vi "Configure Current Limit.vi"(8 "error in (no error)":errorcluster, 10 "Current Limit":dbl, 11 "Manual PSU in":refnum<class "Manual PSU.lvclass">) -> (0 "error out":errorcluster, 3 "Manual PSU out":refnum<class "Manual PSU.lvclass">)   [LabVIEW 2020, in "Manual PSU.lvclass"]
uses:
  Manual PSU.lvclass
  C:/Sandbox/RF Bench/Source Code/WiSpry Test Framework/Instruments/Power Supply/Power Supply.lvclass
  Power Supply.lvclass/Power Supply.ctl
  Power Supply.lvclass
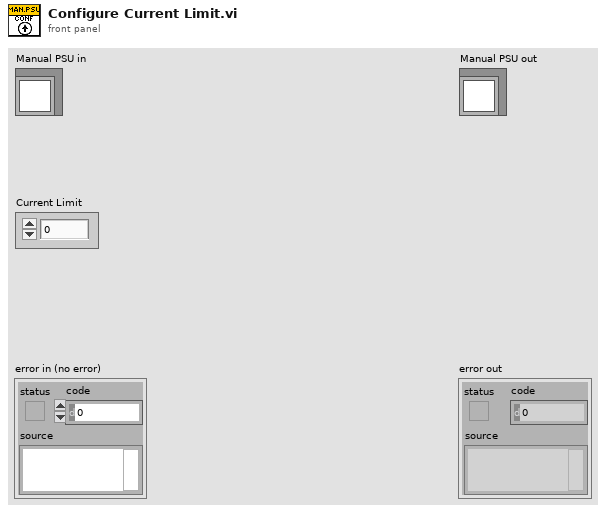
[diagram p1: front panel]
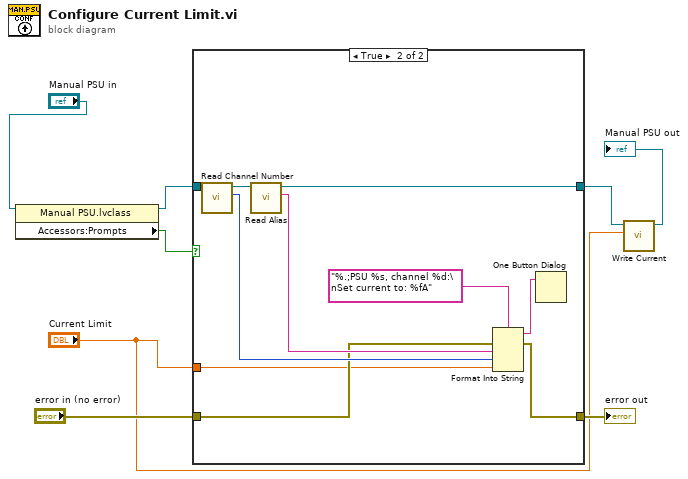
[diagram p0: block diagram]
diagram:
  n1 = property class="Manual PSU.lvclass"(reference="Manual PSU in") -> (reference out=w5:refnum<class "Manual PSU.lvclass">, "Accessors:Prompts"=w4:bool)  [unwired: 1 in, 1 out]
  n2 = case shown="True" w4 {
    tunnel: "error in (no error)" -> [w9 w15]
    tunnel: [w9 w14] -> w7
    tunnel: [w10 w13] -> w2
    tunnel: w5 -> [w10 w12]
    tunnel: "Current Limit" -> [_ w11]
    frame False {
    }
    frame True {
      n3 = call "Read Channel Number.vi"("Power Supply in"=w12) -> ("Channel Number"=w16:u8, "Power Supply out"=w17:refnum<class "Manual PSU.lvclass">)  [unwired: 9 in]
      n4 = call-dynamic "Read Alias.vi"("Power Supply in"=w17) -> ("Alias"=w18:string, "Power Supply out"=w13:refnum<class "Manual PSU.lvclass">)  [unwired: 9 in]
      n5 = Format Into String(format string="%.;PSU %s, channel %d:\nSet current to: %fA", error in=w15, w18, w16, w11) -> (resulting string=w19:string, error out=w14:errorcluster)  [unwired: 1 in]
      n6 = One Button Dialog(message=w19) -> ()  [unwired: 1 in, 1 out]
    }
  }
  "error out" <- w7
  n7 = call "Write Current.vi"("Current"="Current Limit", "Power Supply in"=w2) -> ("Power Supply out"=→"Manual PSU out":refnum<class "Manual PSU.lvclass">)  [unwired: 9 in]
